vi "Configure Local Daq.vi"() -> ()   [LabVIEW 2012]
uses:
  Local Daq Config.ctl
  read-write.ctl
  ini interface.ctl
panel:
  in  "error in":errorcluster
  out "AI.MaxMultiChanRate":dbl
  out "Channels":string
  in  "OK Button":bool
  out "error out":errorcluster
  in  "Local Daq Config":T1={"Sample rate (Hz)"=1.0, "Over sample factor"=1.0, "Terminal Configuration"=enum."Single Ended", "Device"=0, "Max Voltage"=0} {"Max Voltage" items=["1", "1", "2", "2", "4", "5", "10", "20"]; "Device" items=["Dev1"]; "Over sample factor" min=1.0 max=125.0 step=1.0; "Sample rate (Hz)" min=1.0 max=10000.0 step=1.0}
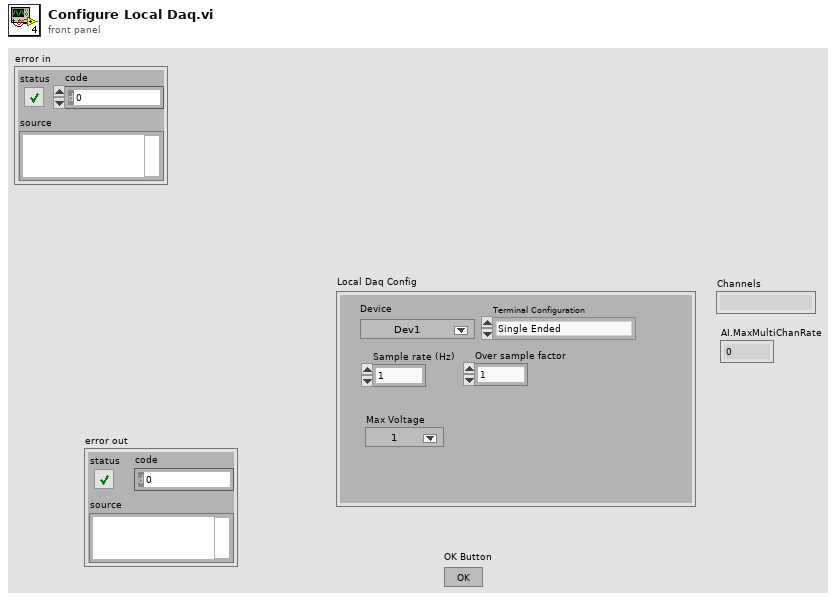
[diagram p1: front panel]
types:
  T1 = typedef "Local Daq Config.ctl" = cluster{"Sample rate (Hz)":dbl, "Over sample factor":dbl, "Terminal Configuration":enum16{"Single Ended", "Differential"}, "Device":u16, "Max Voltage":u16}
  T2 = typedef "ini interface.ctl" = enum16{"dataserver list", "dataserver", "com port", "stamp model", "Local Daq"}
  T3 = typedef "read-write.ctl" = enum16{"read", "write"}
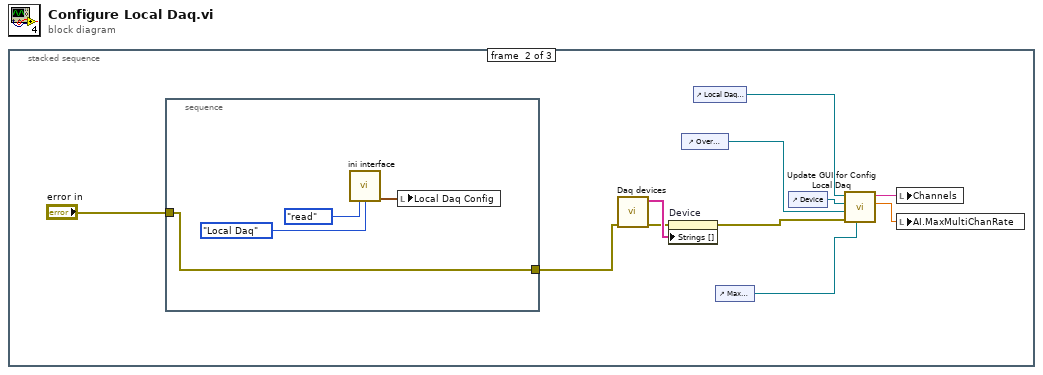
[diagram p0: block diagram]
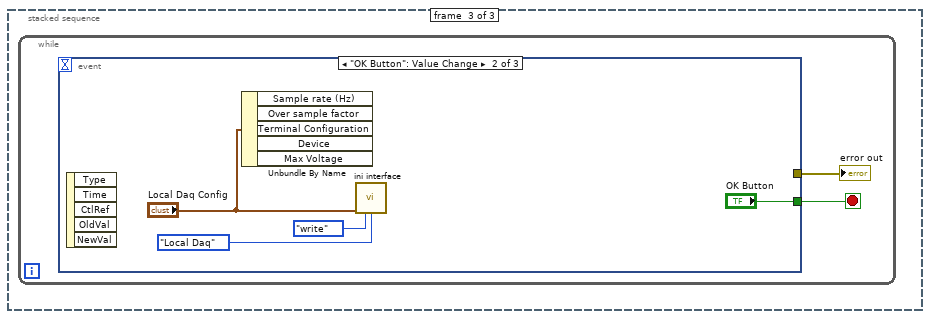
[diagram p3: hidden frame]
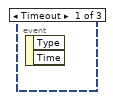
[diagram p4: hidden frame]
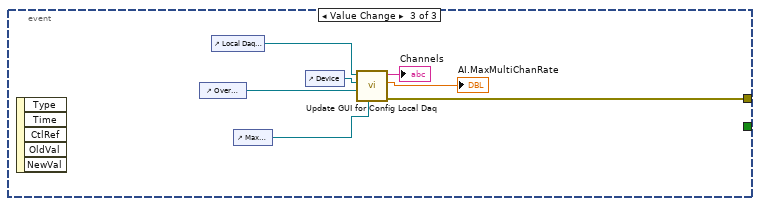
[diagram p5: hidden frame]
diagram:
  n1 = stacked-sequence {
    frame #0 {
    }
    frame #1 {
      n2 = stacked-sequence {
        tunnel: [w12] -> w2
        tunnel: "error in" -> [w12]
        frame #0 {
          n3 = call "ini interface.vi"("direction"=read-write."read", "ini interface"=ini_interface."Local Daq") -> ("Local Daq Config out"=w15:T1)  [unwired: 9 in, 4 out]
          n4 = local write "Local Daq Config"(w15) -> ()
        }
      }
      n5 = call "Daq devices.vi"("error in"=w2) -> ("error out"=w4:errorcluster, "Devices"=w11:string[])  [unwired: 9 in]
      n6 = property on="Device" class="Ring (strict)"(error in=w4, "Strings []"=w11) -> (error out=w3:errorcluster)  [unwired: 1 in, 1 out]
      n7 = control-ref of="Over sample factor"() -> (w7:refnum<vi>)
      n8 = control-ref of="Local Daq Config"() -> (w5:refnum<vi>)
      n9 = control-ref of="Max Voltage"() -> (w6:refnum<vi>)
      n10 = control-ref of="Device"() -> (w8:refnum<vi>)
      n11 = call "Update GUI for Config Local Daq.vi"("Voltage Ring"=w6, "error in (no error)"=w3, "Digital in"=w7, "Ring Refnum"=w8, "Clust Refnum 2"=w5) -> ("AI.MaxMultiChanRate"=w9:dbl, "Channels"=w10:string)  [unwired: 2 in, 3 out]
      n12 = local write "Channels"(w10) -> ()
      n13 = local write "AI.MaxMultiChanRate"(w9) -> ()
    }
    frame #2 {
      n14 = while {
        stop <- w17 stop-if-true
        n15 = event shown="[1] \"OK Button\": Value Change" {
          selector: _ -> [_ _ _]
          dyn-events: _ -> [_ _ _]
          timeout: _ -> [_ _ _]
          tunnel: [_ "OK Button" _] -> w17
          tunnel: [_ _ w26] -> w16
          event Timeout {
            n16 = event-data() -> ()  [unwired: 1 in, 2 out]
          }
          event "OK Button": Value Change {
            n17 = event-data() -> ()  [unwired: 1 in, 5 out]
            n18 = Unbundle By Name("Local Daq Config") -> ()  [unwired: 5 out]
            n19 = call "ini interface.vi"("Local Daq Config"="Local Daq Config", "direction"=read-write."write", "ini interface"=ini_interface."Local Daq") -> ()  [unwired: 8 in, 5 out]
          }
          event Value Change {
            n20 = event-data() -> ()  [unwired: 1 in, 5 out]
            n21 = control-ref of="Over sample factor"() -> (w24:refnum<vi>)
            n22 = control-ref of="Local Daq Config"() -> (w23:refnum<vi>)
            n23 = control-ref of="Max Voltage"() -> (w22:refnum<vi>)
            n24 = control-ref of="Device"() -> (w25:refnum<vi>)
            n25 = call "Update GUI for Config Local Daq.vi"("Voltage Ring"=w22, "Digital in"=w24, "Ring Refnum"=w25, "Clust Refnum 2"=w23) -> ("error out"=w26:errorcluster, "AI.MaxMultiChanRate"=→"AI.MaxMultiChanRate":dbl, "Channels"=→"Channels":string)  [unwired: 3 in, 2 out]
          }
        }
        "error out" <- w16
      }
    }
  }
